vi "Connect Error Controls to Connector Pane.vi"(8 "error in (no error)":errorcluster, 9 "error controls in":cluster{"in":refnum<vi>, "out":refnum<vi>}, 11 "VI in":refnum<vi>) -> (0 "error out":errorcluster, 1 "error controls out":cluster{"in":refnum<vi>, "out":refnum<vi>}, 3 "VI out":refnum<vi>)   [LabVIEW 2017]
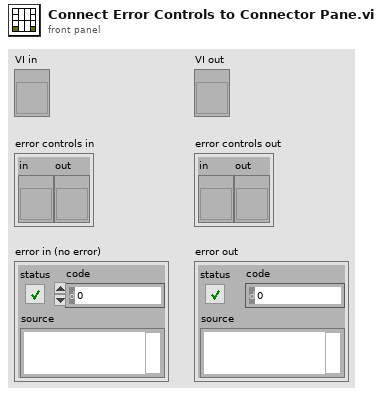
[diagram p1: front panel]
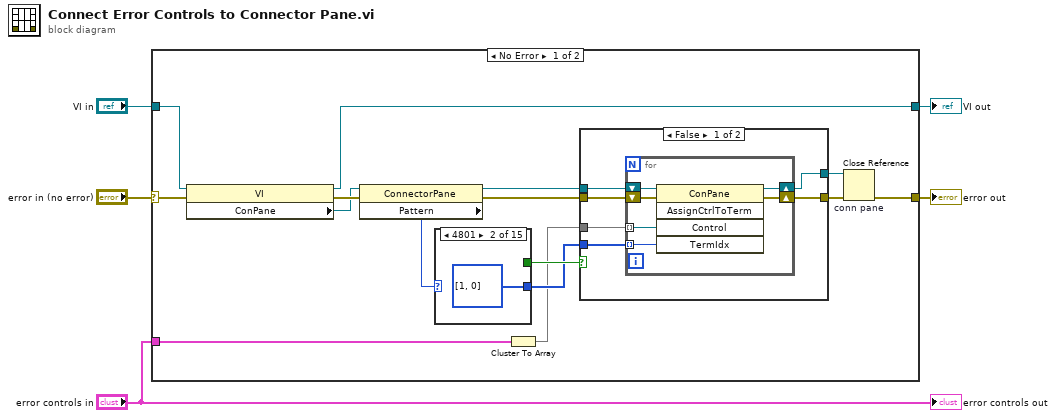
[diagram p0: block diagram]
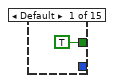
[diagram p3: hidden frame]
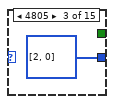
[diagram p4: hidden frame]
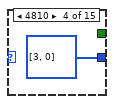
[diagram p5: hidden frame]
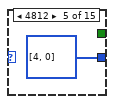
[diagram p6: hidden frame]
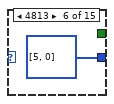
[diagram p7: hidden frame]
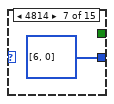
[diagram p8: hidden frame]
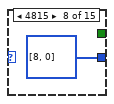
[diagram p9: hidden frame]
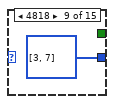
[diagram p10: hidden frame]
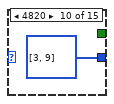
[diagram p11: hidden frame]
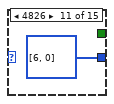
[diagram p12: hidden frame]
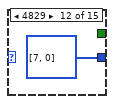
[diagram p13: hidden frame]
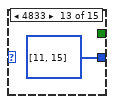
[diagram p14: hidden frame]
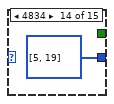
[diagram p15: hidden frame]
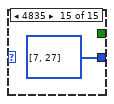
[diagram p16: hidden frame]
diagram:
  n1 = case shown="No Error" "error in (no error)" {
    selector: "error in (no error)" -> [w8 w50]
    tunnel: [w11 w50] -> w5
    tunnel: "VI in" -> [w10 w51]
    tunnel: [w9 w51] -> w3
    tunnel: "error controls in" -> [w7 _]
    frame No Error {
      n2 = property on="Property Node" class="VI"(reference=w10, error in=w8) -> (reference out=w9:refnum<vi>, error out=w16:errorcluster, "ConPane"=w15:refnum<vi>)
      n3 = property on="Property Node" class="ConnectorPane"(reference=w15, error in=w16) -> (reference out=w14:refnum<vi>, error out=w17:errorcluster, "Pattern"=w19:u32)
      n4 = case shown="4801" w19 {
        tunnel: [_ u32[] [1, 0] ("Terminal Index") u32[] [2, 0] ("Terminal Index") u32[] [3, 0] ("Terminal Index") u32[] [4, 0] ("Terminal Index") u32[] [5, 0] ("Terminal Index") u32[] [6, 0] ("Terminal Index") u32[] [8, 0] ("Terminal Index") u32[] [3, 7] ("Terminal Index") u32[] [3, 9] ("Terminal Index") u32[] [6, 0] ("Terminal Index") u32[] [7, 0] ("Terminal Index") u32[] [11, 15] ("Terminal Index") u32[] [5, 19] ("Terminal Index") u32[] [7, 27] ("Terminal Index")] -> w18
        tunnel: [TRUE _ _ _ _ _ _ _ _ _ _ _ _ _ _] -> w20
        frame Default {
        }
        frame 4801 {
        }
        frame 4805 {
        }
        frame 4810 {
        }
        frame 4812 {
        }
        frame 4813 {
        }
        frame 4814 {
        }
        frame 4815 {
        }
        frame 4818 {
        }
        frame 4820 {
        }
        frame 4826 {
        }
        frame 4829 {
        }
        frame 4833 {
        }
        frame 4834 {
        }
        frame 4835 {
        }
      }
      n5 = Cluster To Array(cluster=w7) -> (array=w6:refnum<vi>[])
      n6 = case shown="False" w20 {
        tunnel: w18 -> [w26 _]
        tunnel: w17 -> [w25 w33]
        tunnel: w14 -> [w24 w34]
        tunnel: [w23 w33] -> w13
        tunnel: [w22 w34] -> w12
        tunnel: w6 -> [w21 _]
        frame False {
          n7 = for {
            shift-right: [w31] -> w22
            shift-left: w24 -> [w32]
            shift-right: [w28] -> w23
            shift-left: w25 -> [w30]
            tunnel: w26 -> [w29] mode=indexing
            tunnel: w21 -> [w27] mode=indexing
            n8 = invoke class="ConPane" method="AssignCtrlToTerm"(reference=w32, error in=w30, "Control"=w27, "TermIdx"=w29) -> (reference out=w31:refnum<vi>, error out=w28:errorcluster)  [unwired: 1 in, 3 out]
          }
        }
        frame True {
        }
      }
      n9 = Close Reference "conn pane"(reference=w12, error in (no error)=w13) -> (error out=w11:errorcluster)
    }
    frame Error {
    }
  }
  "error out" <- w5
  "VI out" <- w3
  "error controls out" <- "error controls in"
